vi "LVData_read.vi"(8 "error in (no error)":errorcluster, 11 "LVData in":refnum<class "LVData.lvclass">) -> (0 "error out":errorcluster, 1 "DataArray":dbl[][](array[numeric]), 2 "TimeArray":timestamp[](array[timestamp]), 3 "LVData out":refnum<class "LVData.lvclass">, 5 "Labels":string[](array[string]))   [LabVIEW 2020, in "LVData.lvclass"]
uses:
  LVData.lvclass
  LVData.lvclass/LVData.ctl
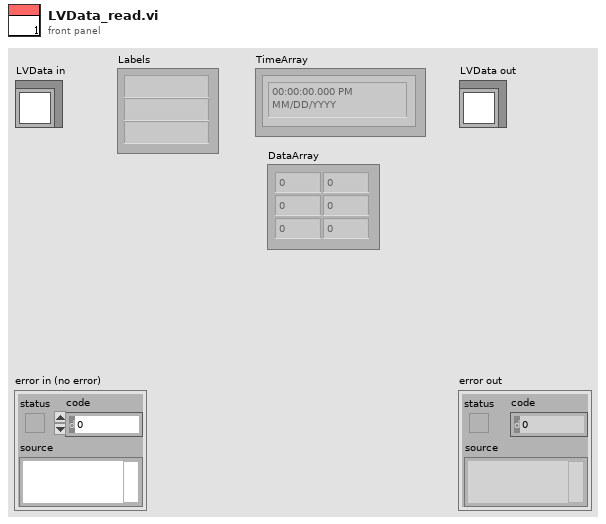
[diagram p1: front panel]
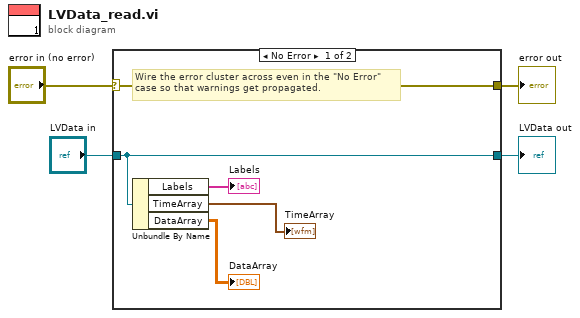
[diagram p0: block diagram]
diagram:
  n1 = case shown="No Error" "error in (no error)" {
    selector: "error in (no error)" -> [w9 w11]
    tunnel: [w9 w11] -> w3
    tunnel: [w8 w10] -> w1
    tunnel: "LVData in" -> [w8 w10]
    frame No Error {
      # "Wire the error cluster across even in the \"No Error\"\ncase so that warnings get propagated."
      n2 = Unbundle By Name(w8) -> ("Labels"=→"Labels":string[], "TimeArray"=→"TimeArray":timestamp[], "DataArray"=→"DataArray":dbl[][])
    }
    frame Error {
    }
  }
  "error out" <- w3
  "LVData out" <- w1
